vi "AttackerStopTactic.vi"(7 "first call":bool, 8 "error in (no error)":errorcluster, 9 "Game in":refnum<class "Game.lvclass">, 10 "Robot":refnum<class "Robot.lvclass">, 11 "AttackerStopTactic in":refnum<class "AttackerStopTactic.lvclass">) -> (0 "error out":errorcluster, 2 "Robot out":refnum<class "Robot.lvclass">, 3 "AttackerStopTactic out":refnum<class "AttackerStopTactic.lvclass">)   [LabVIEW 2018, in "AttackerStopTactic.lvclass"]
uses:
  AttackerStopTactic.lvclass
  Game_class/Game.lvclass
  Robot_class/Robot.lvclass
  C:/Users/Leonardo/Documents/RoboIme/Futebol/SSL/MEXER/SSL_AI/Tactic_class/Tactic.lvclass
  Tactic_class/Tactic.lvclass/Tactic.ctl
  Skillbook_class/Skillbook.lvclass/Skillbook.ctl
  Game_class/Game.lvclass/Game.ctl
  States.ctl
  Robot_class/tactics.ctl
  Utilities_class/Utilities.lvclass
  Parameters_class/Parameters.lvclass/Parameters.ctl
  Object_class/Object.lvclass/Object.ctl
  Robot_class/Robot.lvclass/Robot.ctl
  AttackerStopTactic.lvclass/AttackerStopTactic.ctl
  Game_class/Read Parameters.lvclass.vi
  Parameters_class/Read AttakingOurselves.vi
  Parameters_class/Read DistanceStop.vi
  Game_class/Read BallRef.vi
  Object_class/Read x.vi
  Object_class/Read y.vi
  Game_class/Read FieldRef.vi
  Tactic_class/Read Skillbook.vi
  Skillbook_class/Read AttackerBlockSkill.vi
  Skillbook_class/Read AttackerAimGoalSkill.vi
  Robot_class/Read dest_x.vi
  Robot_class/Read dest_y.vi
  Write States.vi
  Robot_class/Write dest_x.vi
  Robot_class/Write dest_y.vi
  Robot_class/Write tactic.vi
  Ball_class/Ball.lvclass
  C:/Users/Leonardo/Documents/RoboIme/Futebol/SSL/MEXER/SSL_AI/Object_class/Object.lvclass
  Parameters_class/Parameters.lvclass
  Field_class/Field.lvclass
  Skillbook_class/Skillbook.lvclass
  AttackerAimGoalSkill_class/AttackerAimGoalSkill.lvclass
  AttackerBlockSkill_class/AttackerBlockSkill.lvclass
panel:
  out "x .or. y?":bool
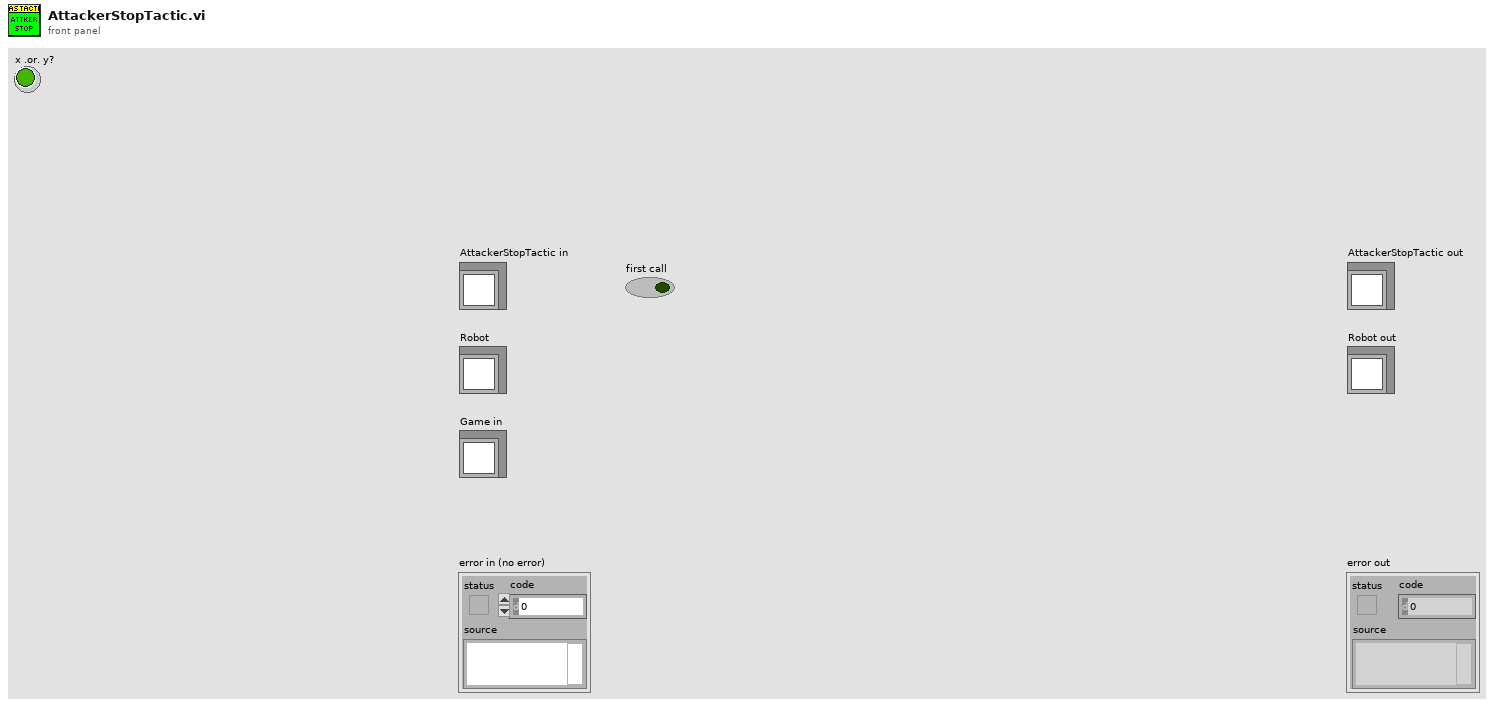
[diagram p1: front panel]
types:
  T1 = typedef "tactics.ctl" = enum16{"PenaltyAttacker", "PassObserver", "PenaltyDefense", "Test", "DefendGoal", "Marker", "FollowAttacker", "DefendArea", "Shoot", "AttackerAimGoal", "AttackerBallOutOfField", "AttackerBlock", "AttackerStop", "Duelist", "Halt", "ZigZag", "GoTo", "Timeout", "KickToPassReceiver", "PositionToReceivePass", "PassReceiver", "WaitPass"}
  T2 = typedef "AttackerStopTactic.lvclass/States.ctl" = enum16{"Block", "AimGoal", "Exit"}
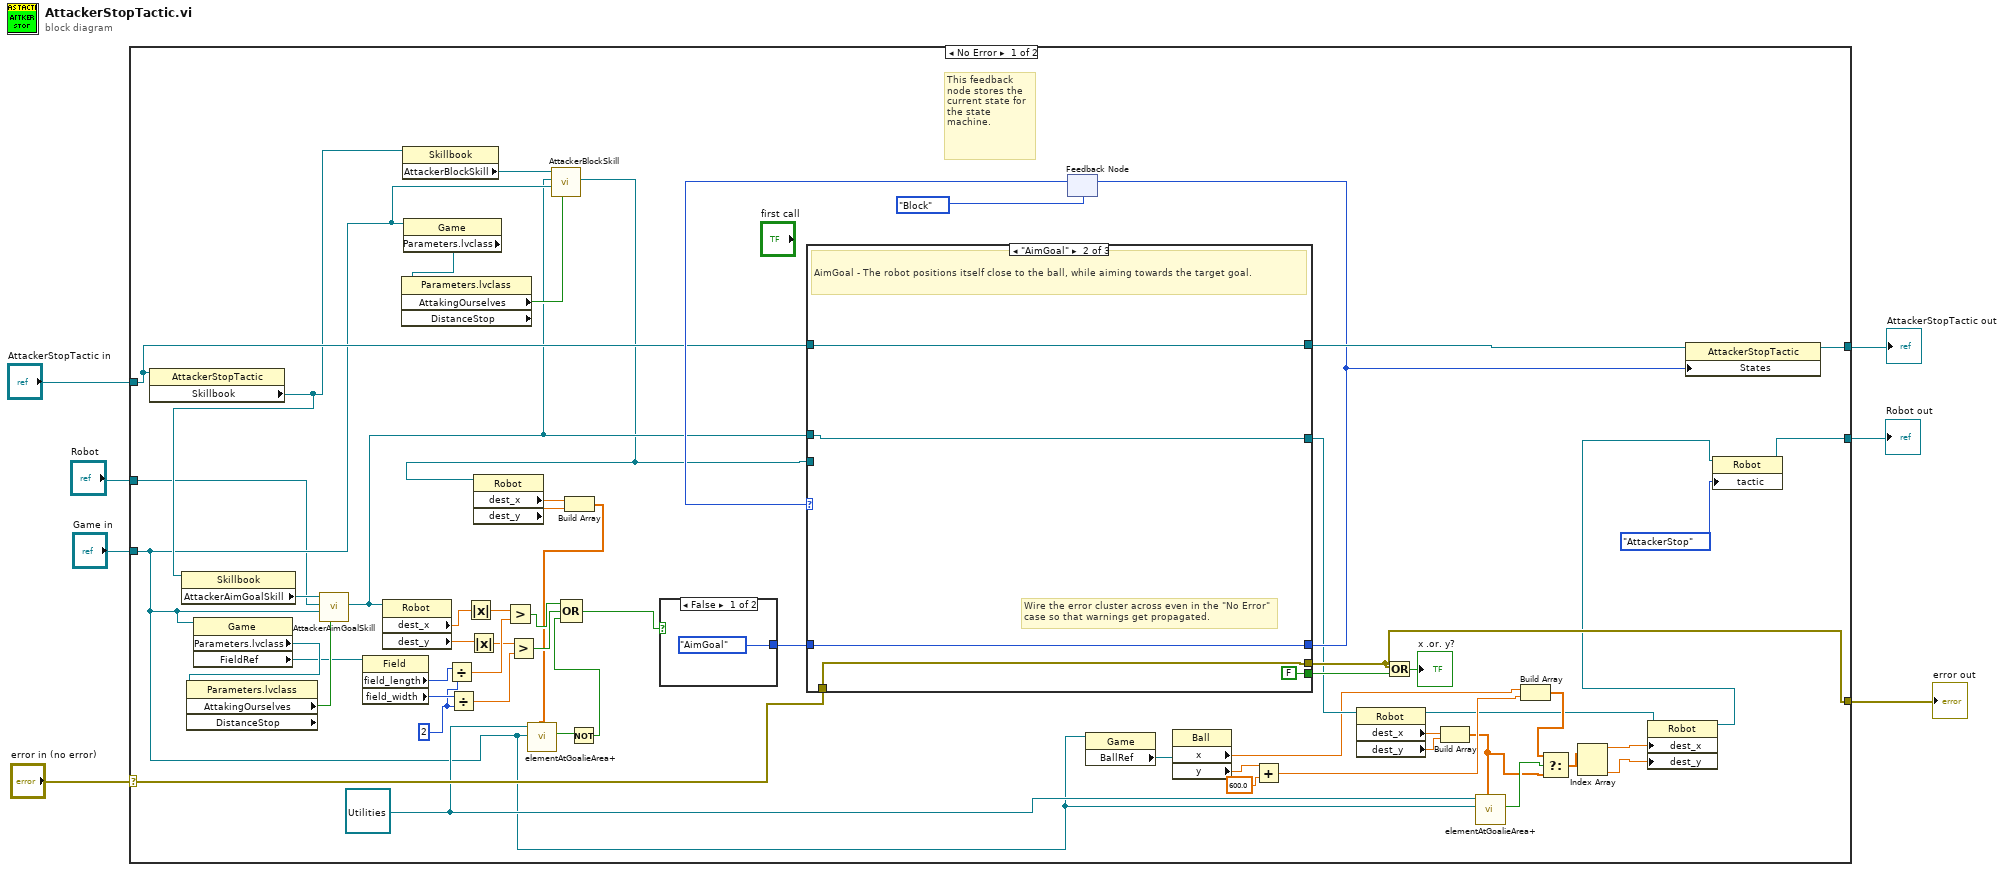
[diagram p0: block diagram]
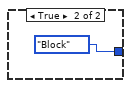
[diagram p2: hidden frame]
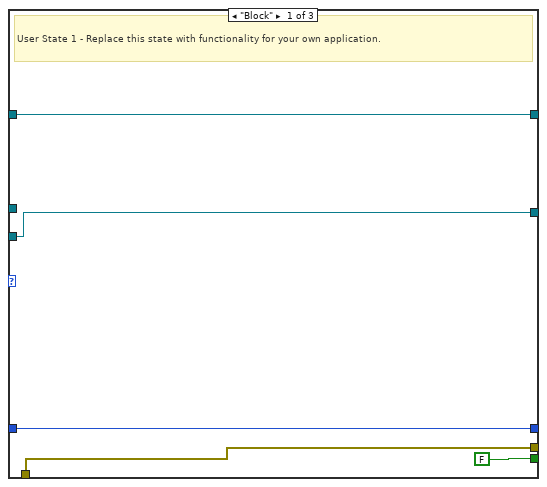
[diagram p3: hidden frame]
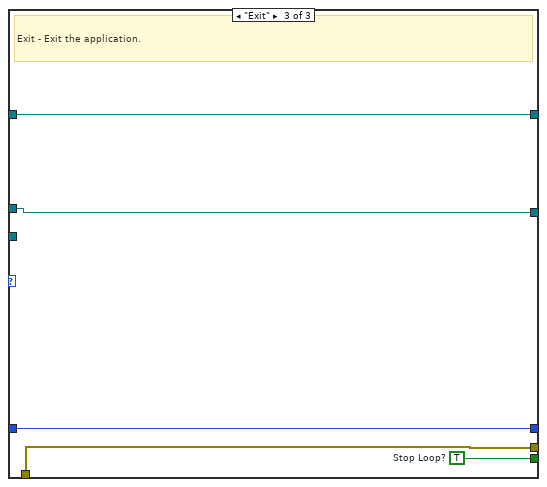
[diagram p4: hidden frame]
diagram:
  n1 = case shown="No Error" "error in (no error)" {
    selector: "error in (no error)" -> [w47 w86]
    tunnel: [w46 w86] -> w6
    tunnel: [w62 w85] -> w4
    tunnel: "AttackerStopTactic in" -> [w61 w85]
    tunnel: "Game in" -> [w14 _]
    tunnel: "Robot" -> [w13 w84]
    tunnel: [w43 w84] -> w1
    frame No Error {
      w34 = refnum<class "Utilities.lvclass"> refnum ("Utilities in")
      w53 = 2 ("y")
      # "This feedback node stores the current state for the state machine."
      # "Wire the error cluster across even in the \"No Error\"\ncase so that warnings get propagated."
      n2 = property class="AttackerStopTactic"(reference=w61) -> ("Skillbook"=w15:refnum<class "Skillbook.lvclass">)  [unwired: 1 in, 2 out]
      n3 = property class="Skillbook"(reference=w15) -> ("AttackerAimGoalSkill"=w59:refnum<class "AttackerAimGoalSkill.lvclass">)  [unwired: 1 in, 2 out]
      n4 = property class="Game"(reference=w14) -> ("Parameters.lvclass"=w58:refnum<class "Parameters.lvclass">, "FieldRef"=w56:refnum<class "Field.lvclass">)  [unwired: 1 in, 2 out]
      n5 = property class="Parameters.lvclass" props=["AttakingOurselves", "DistanceStop"](reference=w58) -> ("AttakingOurselves"=w57:bool)  [unwired: 1 in, 3 out]
      n6 = call-dynamic "AttackerAimGoalSkill.vi"("AttackOurselves"=w57, "Game"=w14, "Robot"=w13, "AttackerAimGoalSkill in"=w59) -> ("Robot out"=w12:refnum<class "Robot.lvclass">)  [unwired: 5 in, 2 out]
      n7 = property class="Field"(reference=w56) -> ("field_length"=w55:i32, "field_width"=w54:i32)  [unwired: 1 in, 2 out]
      n8 = property class="Robot"(reference=w12) -> ("dest_x"=w42:dbl, "dest_y"=w41:dbl)  [unwired: 1 in, 2 out]
      n9 = property class="Skillbook"(reference=w15) -> ("AttackerBlockSkill"=w16:refnum<class "AttackerBlockSkill.lvclass">)  [unwired: 1 in, 2 out]
      n10 = property class="Game"(reference=w14) -> ("Parameters.lvclass"=w17:refnum<class "Parameters.lvclass">)  [unwired: 1 in, 2 out]
      n11 = property class="Parameters.lvclass" props=["AttakingOurselves", "DistanceStop"](reference=w17) -> ("AttakingOurselves"=w18:bool)  [unwired: 1 in, 3 out]
      n12 = Divide(x=w55, y=w53) -> (x/y=w51:dbl)
      n13 = Divide(x=w54, y=w53) -> (x/y=w49:dbl)
      n14 = Absolute Value(x=w42) -> (abs(x)=w52:dbl)
      n15 = Absolute Value(x=w41) -> (abs(x)=w50:dbl)
      n16 = Greater?(x=w52, y=w51) -> (0:w40:bool)
      n17 = Greater?(x=w50, y=w49) -> (0:w39:bool)
      n18 = call-dynamic "AttackerBlockSkill.vi"("AttackOurselves"=w18, "Game"=w14, "Robot"=w12, "AttackerBlockSkill in"=w16) -> ("Robot out"=w11:refnum<class "Robot.lvclass">)  [unwired: 5 in, 2 out]
      n19 = property class="Robot"(reference=w11) -> ("dest_x"=w10:dbl, "dest_y"=w9:dbl)  [unwired: 1 in, 2 out]
      n20 = Build Array(w10, w9) -> (w8:dbl[])
      n21 = call "elementAtGoalieArea+.vi"("Elemento pos."=w8, "Game"=w14, "Utilities in"=w34) -> ("Elemento at goalkeeper area + ?"=w38:bool)  [unwired: 6 in, 2 out]
      n22 = Not(x=w38) -> (.not. x?=w37:bool)
      n23 = Compound Arithmetic op=OR(w40, w39, w37) -> (w36:bool)
      n24 = case shown="False" w36 {
        tunnel: [States."AimGoal" ("States") States."Block" ("States")] -> w48
        frame False {
        }
        frame True {
        }
      }
      n25 = feedback #1(States."Block" ("States")) -> (w64:T2)
      n26 = case shown="\"AimGoal\"" w64 {
        tunnel: [FALSE ("Stop Loop?") FALSE ("Stop Loop?") w83] -> w66
        tunnel: [w69 w77 w81] -> w22
        tunnel: [w72 w76 w82] -> w63
        tunnel: w61 -> [w72 w76 w82]
        tunnel: [w71 w78 w79] -> w45
        tunnel: w48 -> [w71 w78 w79]
        tunnel: w12 -> [_ w77 w81]
        tunnel: [w70 w74 w80] -> w46
        tunnel: w47 -> [w70 w74 w80]
        tunnel: w11 -> [w69 _ _]
        frame "Block" {
          # "User State 1 - Replace this state with functionality for your own application."
        }
        frame "AimGoal" {
          # "AimGoal - The robot positions itself close to the ball, while aiming towards the target goal."
        }
        frame "Exit" {
          w83 = TRUE  # Stop Loop?
          # "Exit - Exit the application."
        }
      }
      n27 = feedback-in #1(w45) -> ()
      n28 = property class="Game"(reference=w14) -> ("BallRef"=w31:refnum<class "Ball.lvclass">)  [unwired: 1 in, 2 out]
      n29 = property class="Ball"(reference=w31) -> ("x"=w20:dbl, "y"=w30:dbl)  [unwired: 1 in, 2 out]
      n30 = Add(x=w30, y=600.0) -> (x+y=w28:dbl)
      n31 = property class="Robot"(reference=w22) -> (reference out=w26:refnum<class "Robot.lvclass">, "dest_x"=w32:dbl, "dest_y"=w35:dbl)  [unwired: 1 in, 1 out]
      n32 = Or(x=w46, y=w66) -> (x .or. y?=→"x .or. y?":bool)
      n33 = Build Array(w32, w35) -> (w19:dbl[])
      n34 = call "elementAtGoalieArea+.vi"("Elemento pos."=w19, "Game"=w14, "Utilities in"=w34) -> ("Elemento at goalkeeper area + ?"=w33:bool)  [unwired: 6 in, 2 out]
      n35 = Build Array(w20, w28) -> (w27:dbl[])
      n36 = Select(t=w27, s=w33, f=w19) -> (s? t:f=w25:dbl[])
      n37 = Index Array(array=w25) -> (element #1=w24:dbl, element #2=w23:dbl)  [unwired: 2 in]
      n38 = property class="Robot"(reference=w26, "dest_x"=w24, "dest_y"=w23) -> (reference out=w21:refnum<class "Robot.lvclass">)  [unwired: 1 in, 1 out]
      n39 = property class="AttackerStopTactic"(reference=w63, "States"=w45) -> (reference out=w62:refnum<class "AttackerStopTactic.lvclass">)  [unwired: 1 in, 1 out]
      n40 = property class="Robot"(reference=w21, "tactic"=tactics."AttackerStop") -> (reference out=w43:refnum<class "Robot.lvclass">)  [unwired: 1 in, 1 out]
    }
    frame Error {
    }
  }
  "error out" <- w6
  "AttackerStopTactic out" <- w4
  "Robot out" <- w1
